vi "Create.vi"(8 "error in (no error)":errorcluster, 11 "Report Ref":refnum<k7>) -> (0 "error out":errorcluster, 3 "Report out":refnum<class "Report.lvclass">)   [LabVIEW 2020, in "TSnax.lvlib" / "Report.lvclass"]
uses:
  Report.lvclass
  Report.lvclass/Report.ctl
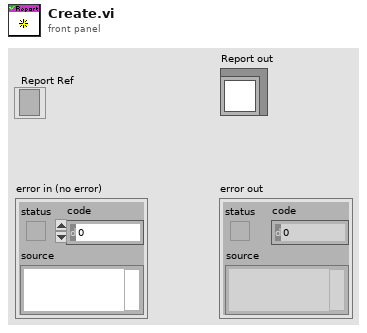
[diagram p1: front panel]
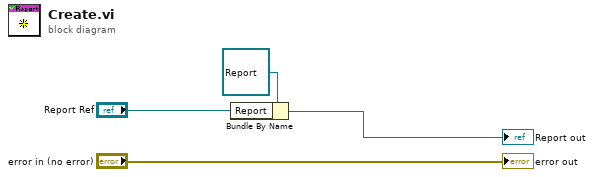
[diagram p0: block diagram]
diagram:
  n1 = Bundle By Name(cluster=refnum<class "Report.lvclass"> refnum ("Report in"), "Report"="Report Ref") -> (→"Report out":refnum<class "Report.lvclass">)
  "error out" <- "error in (no error)"
